vi "DriveImmediate.vi"(6 "SubSystem Data":T9, 8 "error in (no error)":errorcluster, 9 "Control Mode":T8, 10 "Cluster":cluster{"Start Time (ms)":u32, "Iterations":i32}, 11 "RobotDriveRef":T1) -> (0 "error out":errorcluster, 1 "Left Setpoint":dbl, 2 "RobotDriveRef Out":T1, 3 "Wait":dbl, 4 "Right Setpoint":dbl, 5 "Boolean":bool)   [LabVIEW 2015]
uses:
  Drive Setpoints.ctl
  Drive Operations.ctl
  Advanced Drive VIs/RobotDrive Type Def.ctl
  <vilib>/Rock Robotics/WPI/MotorControl/WPI_MotorControlDeviceRef.ctl
  <vilib>/Rock Robotics/WPI/MotorControl/WPI_MotorControlType.ctl
  <vilib>/Rock Robotics/SystemInterfaces/DIO/FPGA_DIOPWMChannel.ctl
  <vilib>/Rock Robotics/WPI/PWM/WPI_PWMDeadband.ctl
  <vilib>/Rock Robotics/WPI/CAN/Jaguar/SubVIs/WPI_CANJaguar_ControlMode.ctl
  <vilib>/Rock Robotics/WPI/CAN/TalonSRX/WPI_CANTalonSRX_APIControlMode.ctl
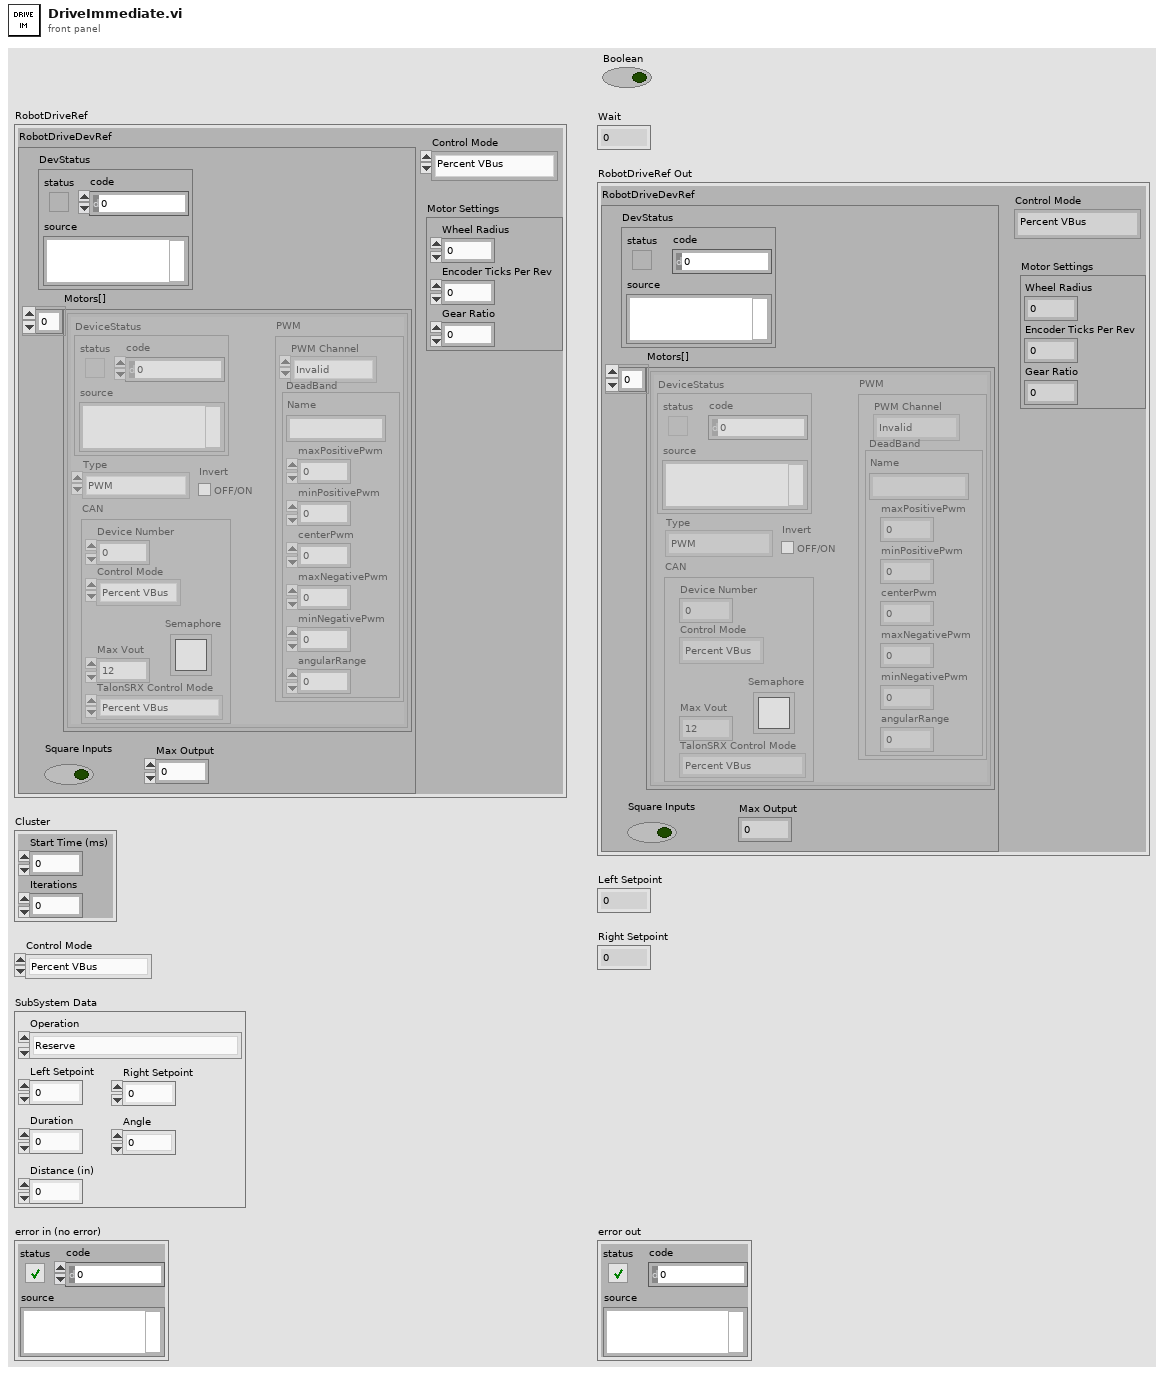
[diagram p1: front panel]
types:
  T1 = typedef "RobotDrive Type Def.ctl" = cluster{"RobotDriveDevRef":cluster{"DevStatus":errorcluster, "Motors[]":T2[], "Square Inputs":bool, "Max Output":dbl}, "Control Mode":T8, "Motor Settings":cluster{"Wheel Radius":dbl, "Encoder Ticks Per Rev":dbl, "Gear Ratio":dbl}}
  T2 = typedef "WPI_MotorControlDeviceRef.ctl" = cluster{"DeviceStatus":errorcluster, "Type":T3, "PWM":cluster{"PWM Channel":T4, "DeadBand":T5}, "CAN":cluster{"Device Number":u8, "Control Mode":T6, "Semaphore":T7, "Max Vout":dbl, "TalonSRX Control Mode":T8}, "Invert":bool}
  T3 = typedef "WPI_MotorControlType.ctl" = enum16{"PWM", "CAN", "CANTalonSRX"}
  T4 = typedef "FPGA_DIOPWMChannel.ctl" = enum8{"PWM 0", "PWM 1", "PWM 2", "PWM 3", "PWM 4", "PWM 5", "PWM 6", "PWM 7", "PWM 8", "PWM 9", "PWM MXP 0", "PWM MXP 1", "PWM MXP 2", "PWM MXP 3", "PWM MXP 4", "PWM MXP 5", "PWM MXP 6", "PWM MXP 7", "PWM MXP 8", "PWM MXP 9", "Invalid"}
  T5 = typedef "WPI_PWMDeadband.ctl" = cluster{"Name":string, "maxPositivePwm":i32, "minPositivePwm":i32, "centerPwm":i32, "maxNegativePwm":i32, "minNegativePwm":i32, "angularRange":u16}
  T6 = typedef "WPI_CANJaguar_ControlMode.ctl" = enum8{"Percent VBus", "Current", "Speed", "Position", "Voltage"}
  T7 = typedef "Semaphore RefNum" = refnum<k1>
  T8 = typedef "WPI_CANTalonSRX_APIControlMode.ctl" = enum8{"Percent VBus", "Speed", "Position", "Slave", "Unchanged / Invalid", "Voltage Compensation", "Current", "Motion Profile"}
  T9 = typedef "Drive Setpoints.ctl" = cluster{"Operation":T10, "Left Setpoint":dbl, "Right Setpoint":dbl, "Duration":dbl, "Angle":dbl, "Distance (in)":dbl}
  T10 = typedef "Drive Operations.ctl" = enum16{"Reserve", "Read Current", "Immediate", "Drive for Time", "Drive for Distance", "Turn Degrees"}
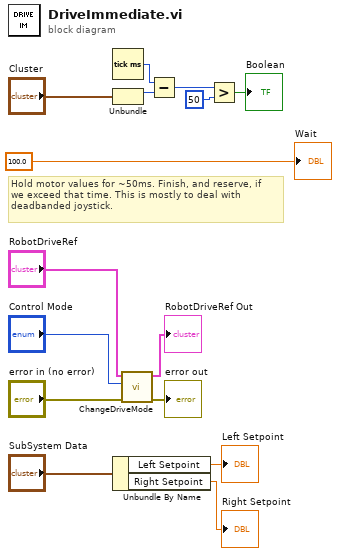
[diagram p0: block diagram]
diagram:
  # "Hold motor values for ~50ms. Finish, and reserve, if\nwe exceed that time. This is mostly to deal with\ndeadbanded joystick."
  n1 = Tick Count (ms)() -> (millisecond timer value=w1:u32)
  n2 = Unbundle("Cluster") -> ("Start Time (ms)"=w5:u32)  [unwired: 1 out]
  n3 = Unbundle By Name("SubSystem Data") -> ("Left Setpoint"=→"Left Setpoint":dbl, "Right Setpoint"=→"Right Setpoint":dbl)
  n4 = call "ChangeDriveMode.vi"("error in (no error)"="error in (no error)", "Control Mode"="Control Mode", "RobotDriveRef"="RobotDriveRef") -> ("error out"=→"error out":errorcluster, "RobotDriveRef Out"=→"RobotDriveRef Out":T1)  [unwired: 7 in]
  n5 = Subtract(x=w1, y=w5) -> (x-y=w4:u32)
  n6 = Greater?(x=w4, y=u8 50 ("Left Motor")) -> (0:→"Boolean":bool)
  "Wait" <- 100.0
